vi "Fetch Multiple Measurements (Voltage Data).vi"(0 "VISA resource name":refnum<visa-resource-name>, 11 "error in (no error)":errorcluster) -> (4 "VISA resource name out":refnum<visa-resource-name>, 6 "Instantaneous Voltage":dbl[](array[numeric]), 8 "Voltage Harmonic Amplitudes":dbl[](array[numeric]), 10 "Voltage Harmonic Phase Angles":dbl[](array[numeric]), 15 "error out":errorcluster)   [LabVIEW 2020, in "Agilent 681x Series.lvlib"]
doc: "Fetches and returns the last 4096 instantaneous voltage measurements, the first 50 harmonic amplitudes and phase values.\n\n<B>Note:</B>\n\nUse this VI only with other low-level VIs. The high-level VIs automatically incorporate this functionality. This VI does not check the instrument status. If you want to check the instrument status, call the Error Query VI at the conclusion of the sequence."
uses:
  <instrlib>/Agilent 681x Series/Agilent 681x Series.lvlib
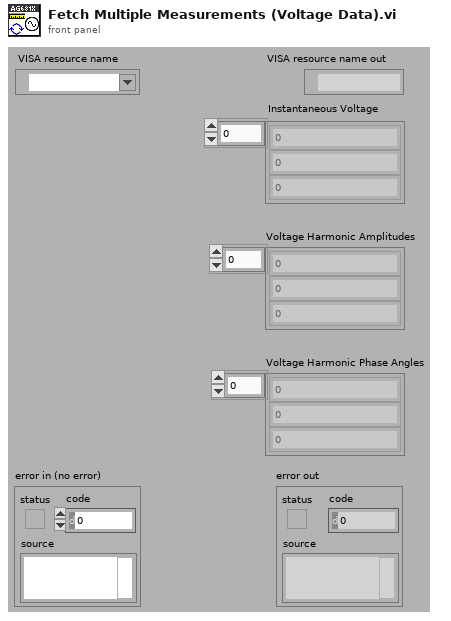
[diagram p1: front panel]
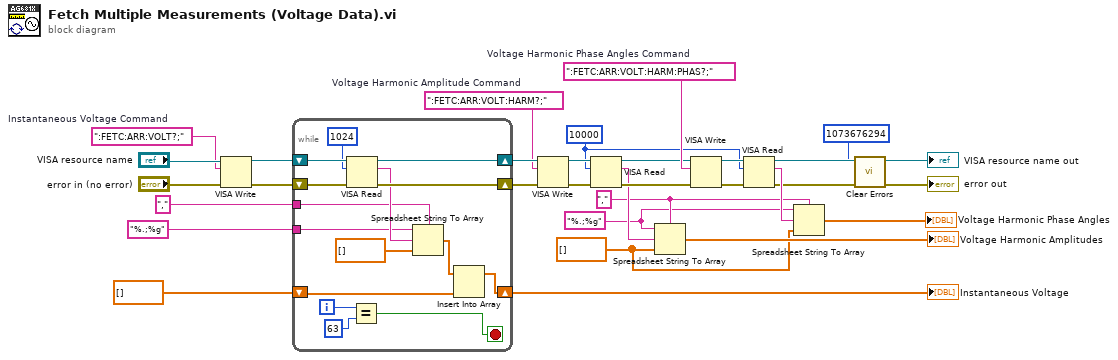
[diagram p0: block diagram]
diagram:
  w2 = dbl[] []
  w5 = "," ("format string")
  w3 = "%.;%g" ("format string")
  w14 = u32 10000 ("byte count")
  w21 = ":FETC:ARR:VOLT:HARM:PHAS?;"  # Voltage Harmonic Phase Angles Command
  w13 = ":FETC:ARR:VOLT:HARM?;"  # Voltage Harmonic Amplitude Command
  w27 = ":FETC:ARR:VOLT?;"  # Instantaneous Voltage Command
  n1 = VISA Write(VISA resource name="VISA resource name", write buffer=w27, error in (no error)="error in (no error)") -> (VISA resource name out=w28:refnum<visa-resource-name>, error out=w29:errorcluster)  [unwired: 1 out]
  n2 = while {
    tunnel: "," ("format string") -> [w39]
    tunnel: "%.;%g" ("format string") -> [w38]
    shift-right: [w44] -> w26
    shift-left: w29 -> [w46]
    shift-right: [w43] -> w22
    shift-left: w28 -> [w45]
    shift-right: [w35] -> w12
    shift-left: dbl[] [] -> [w36]
    i -> [w34]
    stop <- w32 stop-if-true
    n3 = VISA Read(VISA resource name=w45, byte count=u32 1024, error in (no error)=w46) -> (VISA resource name out=w43:refnum<visa-resource-name>, read buffer=w40:string, error out=w44:errorcluster)  [unwired: 1 out]
    n4 = Equal?(x=w34, y=63) -> (x = y?=w32:bool)
    n5 = Spreadsheet String To Array(delimiter (Tab)=w39, format string=w38, spreadsheet string=w40, array type (2D Dbl)=dbl[] []) -> (array=w37:dbl[])
    n6 = Insert Into Array(array=w37, new element=w36) -> (w35:dbl[])  [unwired: 1 in]
  }
  "Instantaneous Voltage" <- w12
  n7 = VISA Write(VISA resource name=w22, write buffer=w13, error in (no error)=w26) -> (VISA resource name out=w20:refnum<visa-resource-name>, error out=w24:errorcluster)  [unwired: 1 out]
  n8 = VISA Read(VISA resource name=w20, byte count=w14, error in (no error)=w24) -> (VISA resource name out=w19:refnum<visa-resource-name>, read buffer=w16:string, error out=w25:errorcluster)  [unwired: 1 out]
  n9 = Spreadsheet String To Array(delimiter (Tab)=w5, format string=w3, spreadsheet string=w16, array type (2D Dbl)=w2) -> (array=→"Voltage Harmonic Amplitudes":dbl[])
  n10 = VISA Write(VISA resource name=w19, write buffer=w21, error in (no error)=w25) -> (VISA resource name out=w18:refnum<visa-resource-name>, error out=w23:errorcluster)  [unwired: 1 out]
  n11 = VISA Read(VISA resource name=w18, byte count=w14, error in (no error)=w23) -> (VISA resource name out=→"VISA resource name out":refnum<visa-resource-name>, read buffer=w15:string, error out=w8:errorcluster)  [unwired: 1 out]
  n12 = Spreadsheet String To Array(delimiter (Tab)=w5, format string=w3, spreadsheet string=w15, array type (2D Dbl)=w2) -> (array=→"Voltage Harmonic Phase Angles":dbl[])
  n13 = call <vilib>:"Clear Errors.vi"("error in (no error)"=w8, "specific error code to clear (0: all)"=1073676294) -> ("error out"=→"error out":errorcluster)  [unwired: 4 in, 1 out]
